vi "KE2000 Read.vi"(8 "error in (no error)":errorcluster, 9 "Read?":bool=TRUE, 10 "Setup?":bool, 11 "VISA resource name":refnum<visa-resource-name>) -> (0 "error out":errorcluster, 2 "uA":string, 3 "VISA resource name out":refnum<visa-resource-name>)   [LabVIEW 2017]
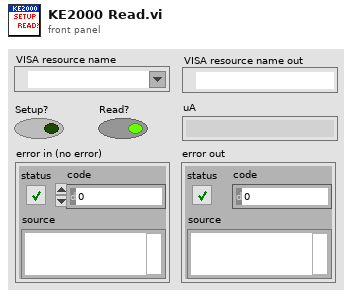
[diagram p1: front panel]
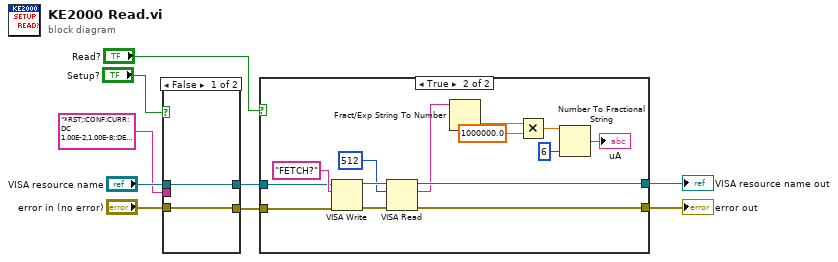
[diagram p0: block diagram]
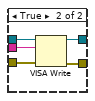
[diagram p3: hidden frame]
diagram:
  n1 = case shown="False" "Setup?" {
    tunnel: [w10 w16] -> w7
    tunnel: [w11 w15] -> w6
    tunnel: "VISA resource name" -> [w11 w14]
    tunnel: "error in (no error)" -> [w10 w13]
    tunnel: "*RST;:CONF:CURR:DC 1.00E-2,1.00E-8;:DET:BAND 20;:ZERO:AUTO OFF;:INP:IMP:AUTO OFF;" ("write buffer") -> [_ w12]
    frame False {
    }
    frame True {
      n2 = VISA Write(VISA resource name=w14, write buffer=w12, error in (no error)=w13) -> (VISA resource name out=w15:refnum<visa-resource-name>, error out=w16:errorcluster)  [unwired: 1 out]
    }
  }
  n3 = case shown="True" "Read?" {
    tunnel: [w17 w32] -> w9
    tunnel: [w18 w31] -> w8
    tunnel: w7 -> [w17 w20]
    tunnel: w6 -> [w18 w19]
    frame False {
    }
    frame True {
      n4 = VISA Write(VISA resource name=w19, write buffer="FETCH?", error in (no error)=w20) -> (VISA resource name out=w30:refnum<visa-resource-name>, error out=w29:errorcluster)  [unwired: 1 out]
      n5 = VISA Read(VISA resource name=w30, byte count=u32 512, error in (no error)=w29) -> (VISA resource name out=w31:refnum<visa-resource-name>, read buffer=w26:string, error out=w32:errorcluster)  [unwired: 1 out]
      n6 = Fract/Exp String To Number(string=w26) -> (number=w25:dbl)  [unwired: 3 in, 1 out]
      n7 = Multiply(x=w25, y=1000000.0) -> (x*y=w23:dbl)
      n8 = Number To Fractional String(number=w23, precision (6)=i16 6) -> (F-format string=→"uA":string)  [unwired: 2 in]
    }
  }
  "error out" <- w9
  "VISA resource name out" <- w8
